vi "Clear buffer.vi"(4 "Error in":errorcluster, 6 "dt for timeout (ms)":u32, 7 "VISA resource name in":refnum<visa-resource-name>) -> (0 "Error out":errorcluster, 3 "VISA resource name out":refnum<visa-resource-name>)   [LabVIEW 2015]
panel:
  out "n Loops":i32
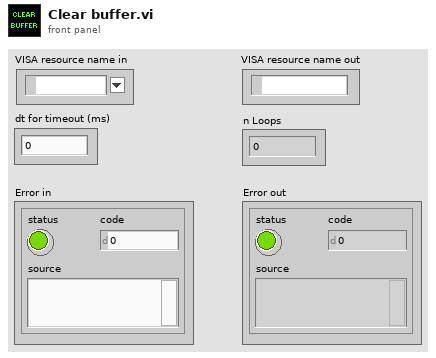
[diagram p1: front panel]
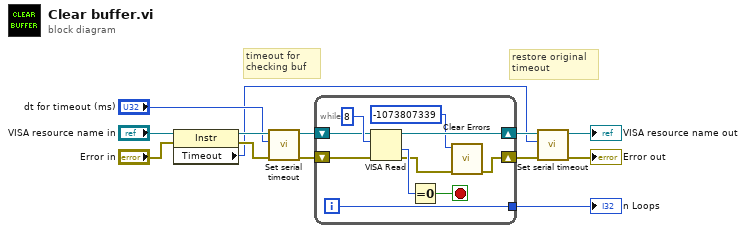
[diagram p0: block diagram]
diagram:
  # "timeout for checking buf"
  # "restore original timeout"
  n1 = property class="Instr"(reference="VISA resource name in", error in="Error in") -> (reference out=w10:refnum<visa-resource-name>, error out=w9:errorcluster, "Timeout"=w1:u32)
  n2 = call "Set serial timeout.vi"("Error in"=w9, "timeout (ms)"="dt for timeout (ms)", "VISA resource name"=w10) -> ("Error out"=w8:errorcluster, "VISA resource name out"=w7:refnum<visa-resource-name>)  [unwired: 7 in]
  n3 = while {
    shift-right: [w15] -> w4
    shift-left: w8 -> [w21]
    shift-right: [w20] -> w5
    shift-left: w7 -> [w22]
    tunnel: [w14] -> w13
    i -> [w14]
    stop <- w18 stop-if-true
    n4 = VISA Read(VISA resource name=w22, byte count=u32 8, error in (no error)=w21) -> (VISA resource name out=w20:refnum<visa-resource-name>, return count=w19:u32, error out=w16:errorcluster)  [unwired: 1 out]
    n5 = Equal To 0?(x=w19) -> (x = 0?=w18:bool)
    n6 = call <vilib>:"Clear Errors.vi"("error in (no error)"=w16, "specific error code to clear (0: all)"=-1073807339) -> ("error out"=w15:errorcluster)  [unwired: 4 in, 1 out]
  }
  "n Loops" <- w13
  n7 = call "Set serial timeout.vi"("Error in"=w4, "timeout (ms)"=w1, "VISA resource name"=w5) -> ("Error out"=→"Error out":errorcluster, "VISA resource name out"=→"VISA resource name out":refnum<visa-resource-name>)  [unwired: 7 in]
